vi "Server_Refresh Remote Data.vi"(8 "error in":errorcluster, 11 "Index":i32) -> (0 "error out":errorcluster, 3 "Image":T1, 5 "User Data":T2)   [LabVIEW 2018, in "Cloud Server.lvlib"]
uses:
  Cloud Server.lvlib
  <vilib>/vision/Image Controls.llb/IMAQ Image.ctl
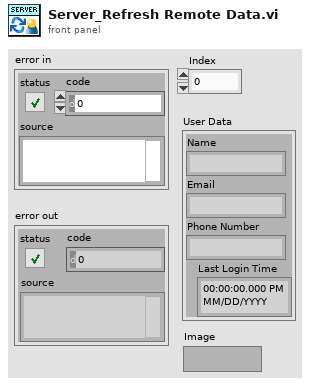
[diagram p1: front panel]
types:
  T1 = typedef "IMAQ Image.ctl" = refnum<image>
  T2 = cluster{"Name":string, "Email":string, "Phone Number":string, "Last Login Time":timestamp}
  T3 = typedef "Cloud Server.lvlib/Server_Connection Properties.ctl" = cluster{"User Data":T4, "Data":waveform(dbl)}
  T4 = typedef "User Data.ctl" = cluster{"Name":string, "Email":string, "Phone Number":string, "User Picture":u32[][], "Last Login Time":timestamp}
  T5 = typedef "Cloud Server.lvlib/Server_Main Data.ctl" = cluster{"Main VI Ref.":refnum<vi>, "Listener ID":refnum<k5>, "Meta data":T6[], "Main Queue":T8, "User Picture":T1}
  T6 = typedef "stm_MetaElement.ctl" = cluster{"Name":T7}
  T7 = typedef "stm_MetaDataElement.ctl" = string
  T8 = typedef "Cloud Server.lvlib/Server_Main Queue.ctl" = cluster{"Server Write Queue":refnum<queue>, "Main Loop Queue":refnum<queue>}
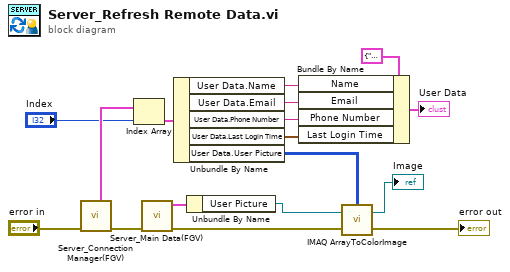
[diagram p0: block diagram]
diagram:
  n1 = call "Server_Connection Manager(FGV).vi"("error in"="error in") -> ("error out"=w5:errorcluster, "All Connection Properties"=w10:T3[])  [unwired: 6 in, 3 out]
  n2 = Index Array(array=w10, index="Index") -> (element=w16:T3)
  n3 = call "Server_Main Data(FGV).vi"("error in"=w5) -> ("error out"=w3:errorcluster, "Main Data Out"=w4:T5)  [unwired: 9 in]
  n4 = Unbundle By Name(w16) -> ("User Data.Name"=w14:string, "User Data.Email"=w13:string, "User Data.Phone Number"=w12:string, "User Data.Last Login Time"=w11:timestamp, "User Data.User Picture"=w7:u32[][])
  n5 = Unbundle By Name(w4) -> ("User Picture"=w2:T1)
  n6 = Bundle By Name(cluster=T2 {"Name"="", "Email"="", "Phone Number"="", "Last Login Time"=timestamp(0 s since 1904-01-01)} ("User Data"), "Name"=w14, "Email"=w13, "Phone Number"=w12, "Last Login Time"=w11) -> (→"User Data":T2)
  n7 = call "IMAQ ArrayToColorImage"("Image Pixels (U32)"=w7, "Image"=w2, "error in (no error)"=w3) -> ("Image Out"=→"Image":T1, "error out"=→"error out":errorcluster)  [unwired: 2 in]
